vi "DataXML example.vi"() -> ()   [LabVIEW 2018]
uses:
  DataXML.lvclass
panel:
  in  "XML file path":path
  out "XML":string
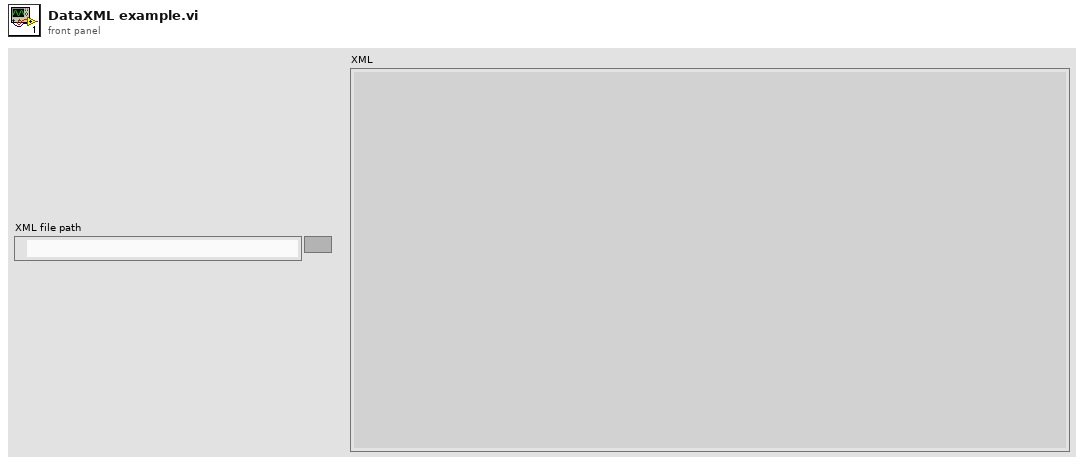
[diagram p1: front panel]
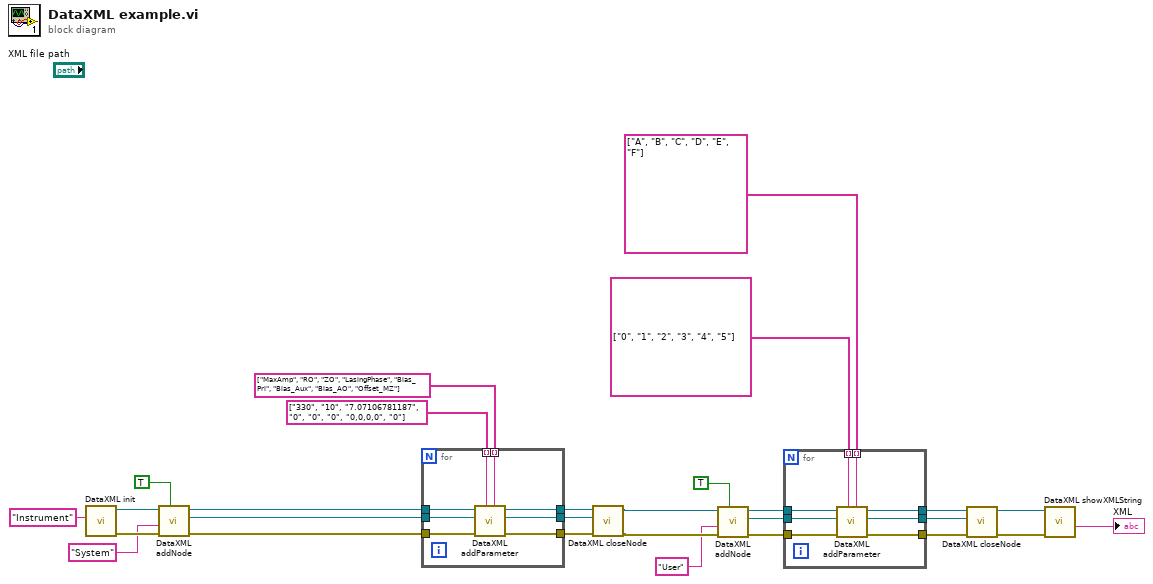
[diagram p0: block diagram]
diagram:
  n1 = call "DataXML init.vi"("root node name"="Instrument") -> ("error out"=w26:errorcluster, "DataXML out"=w27:refnum<class "DataXML.lvclass">)  [unwired: 9 in]
  n2 = call "DataXML addNode.vi"("add_root? (F)"=TRUE, "error in (no error)"=w26, "add tag name"="System", "DataXML in"=w27) -> ("error out"=w21:errorcluster, "new element"=w22:refnum<k20>, "DataXML out"=w23:refnum<class "DataXML.lvclass">)  [unwired: 5 in]
  n3 = for {
    tunnel: string[] ["330", "10", "7.07106781187", "0", "0", "0", "0,0,0,0", "0"] -> [w36] mode=indexing
    tunnel: string[] ["MaxAmp", "RO", "ZO", "LasingPhase", "Bias_Pri", "Bias_Aux", "Bias_AO", "Offset_MZ"] -> [w35] mode=indexing
    tunnel: w23 -> [w34]
    tunnel: w22 -> [w33]
    tunnel: w21 -> [w32]
    tunnel: [w31] -> w20
    tunnel: [w30] -> w19
    tunnel: [w29] -> w18
    n4 = call "DataXML addParameter.vi"("param name"=w35, "param value"=w36, "error in (no error)"=w32, "tag node in"=w33, "DataXML in"=w34) -> ("error out"=w29:errorcluster, "tag node out"=w30:refnum<k20>, "DataXML out"=w31:refnum<class "DataXML.lvclass">)  [unwired: 4 in]
  }
  n5 = call "DataXML closeNode.vi"("error in (no error)"=w18, "tag node"=w19, "DataXML in"=w20) -> ("error out"=w14:errorcluster, "DataXML out"=w15:refnum<class "DataXML.lvclass">)  [unwired: 7 in]
  n6 = call "DataXML addNode.vi"("add_root? (F)"=TRUE, "error in (no error)"=w14, "add tag name"="User", "DataXML in"=w15) -> ("error out"=w10:errorcluster, "new element"=w11:refnum<k20>, "DataXML out"=w12:refnum<class "DataXML.lvclass">)  [unwired: 5 in]
  n7 = for {
    tunnel: string[] ["0", "1", "2", "3", "4", "5"] -> [w44] mode=indexing
    tunnel: string[] ["A", "B", "C", "D", "E", "F"] -> [w43] mode=indexing
    tunnel: w12 -> [w42]
    tunnel: w11 -> [w41]
    tunnel: w10 -> [w40]
    tunnel: [w39] -> w9
    tunnel: [w38] -> w8
    tunnel: [w37] -> w7
    n8 = call "DataXML addParameter.vi"("param name"=w43, "param value"=w44, "error in (no error)"=w40, "tag node in"=w41, "DataXML in"=w42) -> ("error out"=w37:errorcluster, "tag node out"=w38:refnum<k20>, "DataXML out"=w39:refnum<class "DataXML.lvclass">)  [unwired: 4 in]
  }
  n9 = call "DataXML closeNode.vi"("error in (no error)"=w7, "tag node"=w8, "DataXML in"=w9) -> ("error out"=w5:errorcluster, "DataXML out"=w6:refnum<class "DataXML.lvclass">)  [unwired: 7 in]
  n10 = call "DataXML showXMLString.vi"("error in (no error)"=w5, "DataXML in"=w6) -> ("XML"=→"XML":string)  [unwired: 6 in, 3 out]
